vi "Project Test 1.vi"() -> ()   [LabVIEW 2022 SP3]
panel:
  out "Warning Lights":bool[](array[boolean])
  in  "STOP":bool
  out "Boom gate closed if ≠ 0":dbl
  in  "Sensor 2":bool
  in  "Sensor 1":bool
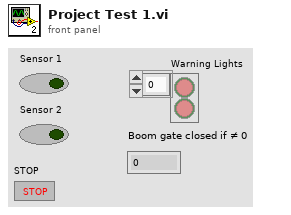
[diagram p1: front panel]
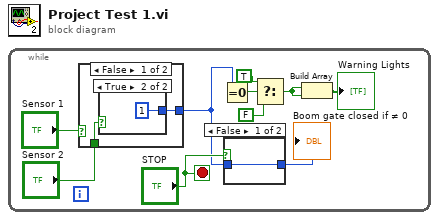
[diagram p0: block diagram]
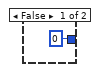
[diagram p2: hidden frame]
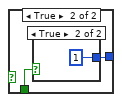
[diagram p3: hidden frame]
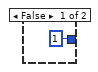
[diagram p4: hidden frame]
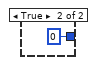
[diagram p5: hidden frame]
diagram:
  n1 = while {
    stop <- "STOP" stop-if-true
    n2 = case shown="False" "Sensor 1" {
      tunnel: "Sensor 2" -> [w11 w16]
      tunnel: [w12 w15] -> w4
      frame False {
        n3 = case shown="True" w11 {
          tunnel: [0 1] -> w12
          frame False {
          }
          frame True {
          }
        }
      }
      frame True {
        n4 = case shown="True" w16 {
          tunnel: [1 1] -> w15
          frame False {
          }
          frame True {
          }
        }
      }
    }
    n5 = Equal To 0?(x=w4) -> (x = 0?=w10:bool)
    n6 = case shown="False" "STOP" {
      tunnel: [w19 0] -> w3
      tunnel: w4 -> [w19 _]
      frame False {
      }
      frame True {
      }
    }
    "Boom gate closed if ≠ 0" <- w3
    n7 = Select(t=TRUE, s=w10, f=FALSE) -> (s? t:f=w1:bool)
    n8 = Build Array(w1, w1) -> (→"Warning Lights":bool[])
  }
